vi "Sort.vi"(11 "ProgramData":T1={"Tytuły"=[], "Folder"=path "", "Data/tytul"=[], "Ostatni index"=-10, "Title"="", "Note"=""}) -> (3 "ProgramData Exit":T1={"Tytuły"=[], "Folder"=path "", "Data/tytul"=[], "Ostatni index"=-10, "Title"="", "Note"=""})   [LabVIEW 2020]
uses:
  #typeDef_ProgramData.ctl
panel:
  in  "D.Rosnąco":bool
  in  "D.Malejąco":bool
  in  "N.Rosnąco":bool
  in  "N.Malejąco":bool
  # "Sort"
  # "By name"
  # "By date"
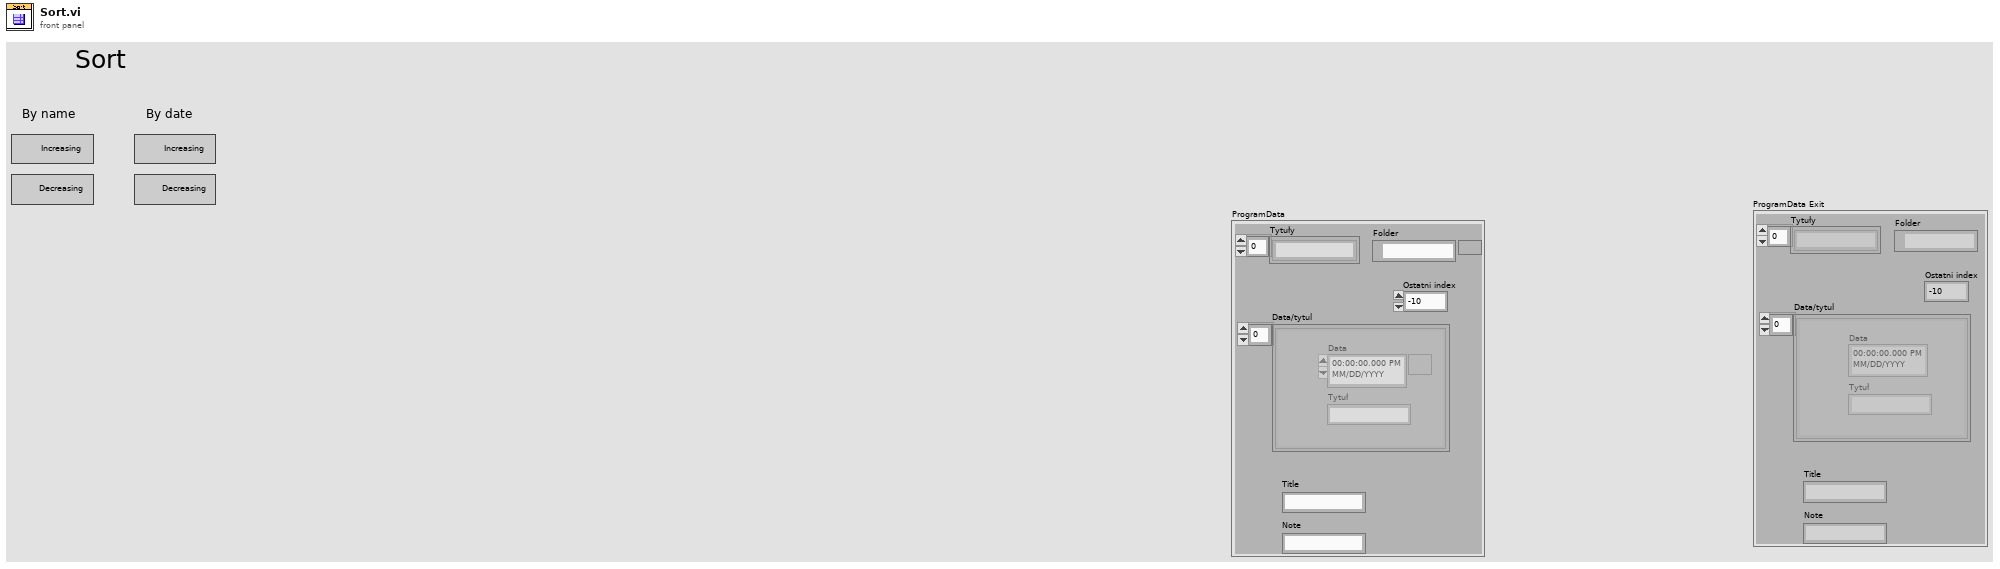
[diagram p1: front panel]
types:
  T1 = typedef "#typeDef_ProgramData.ctl" = cluster{"Tytuły":string[], "Folder":path, "Data/tytul":cluster{"Data":timestamp, "Tytuł":string}[], "Ostatni index":i32, "Title":string, "Note":string}
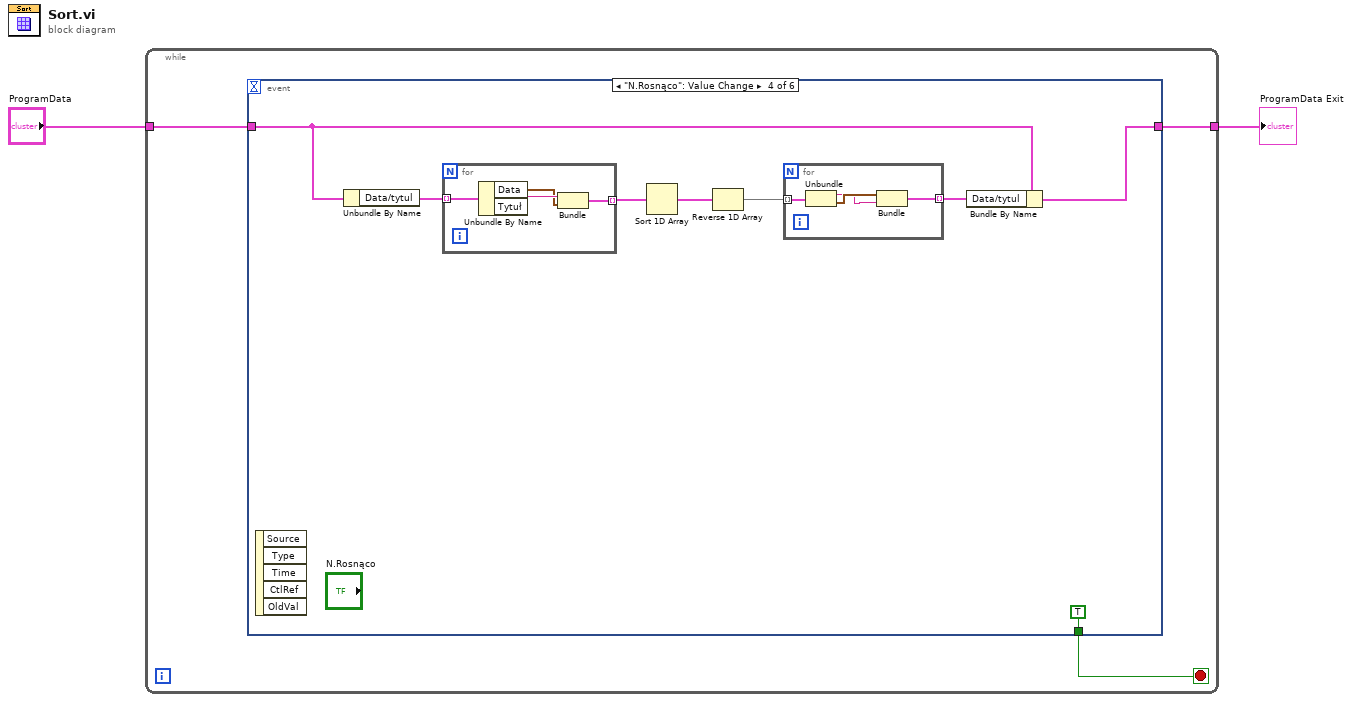
[diagram p0: block diagram]
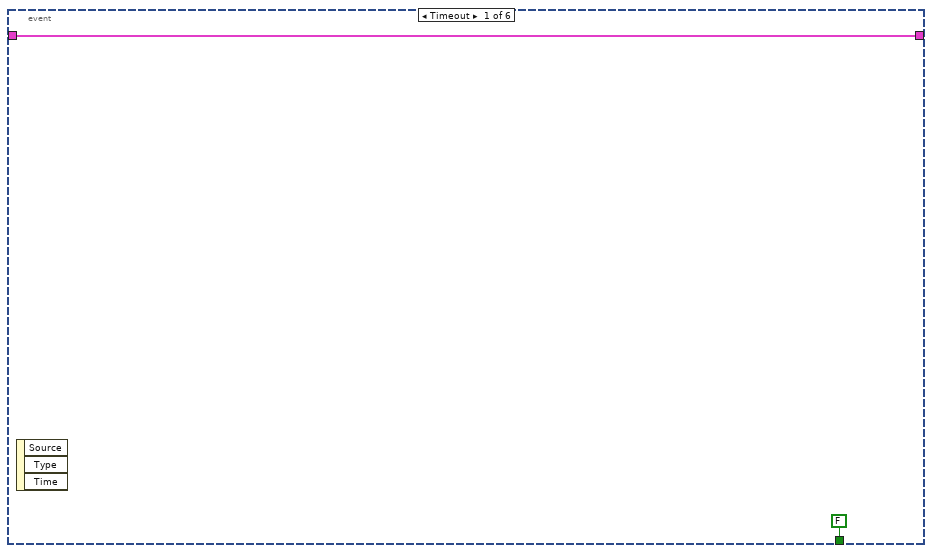
[diagram p2: hidden frame]
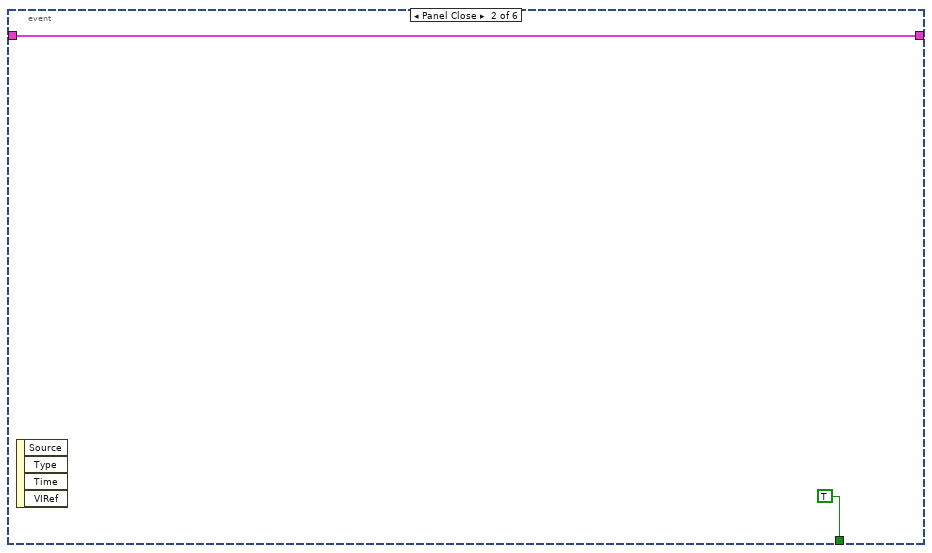
[diagram p3: hidden frame]
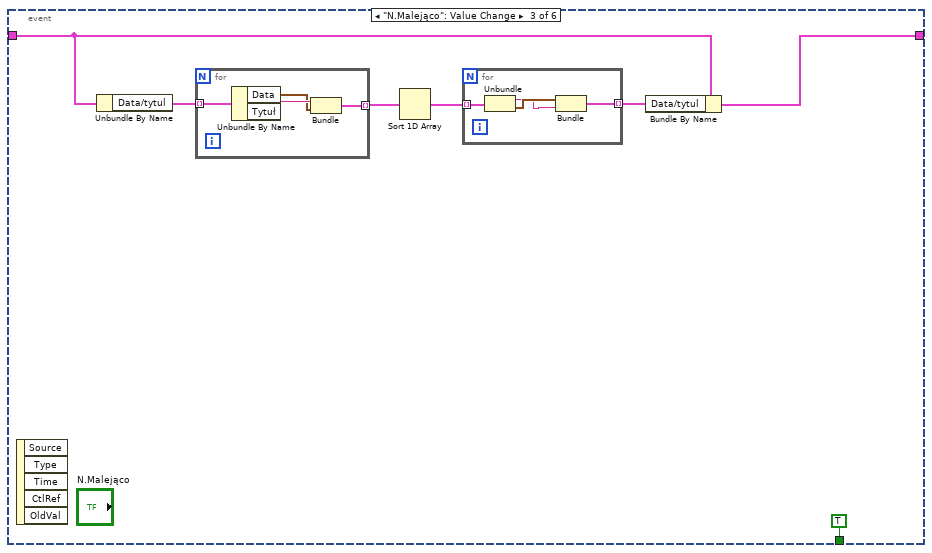
[diagram p4: hidden frame]
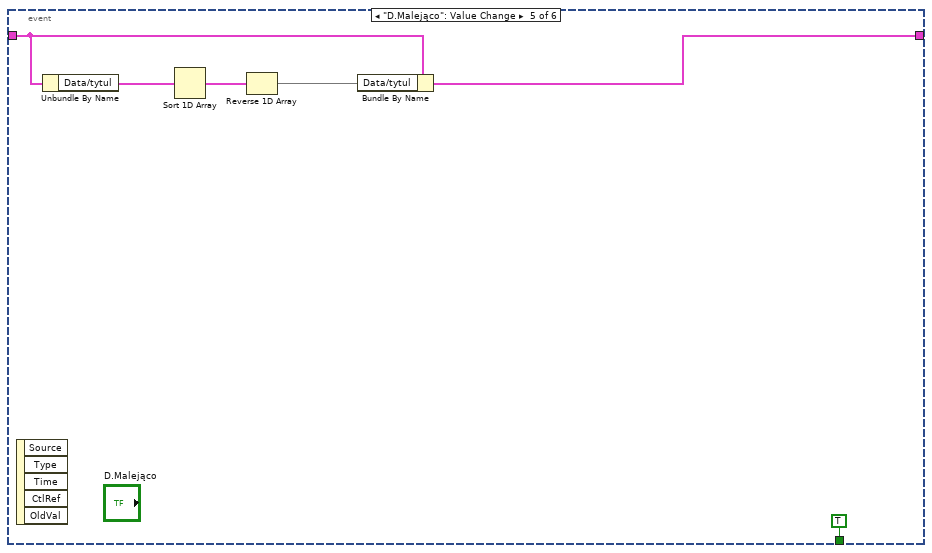
[diagram p5: hidden frame]
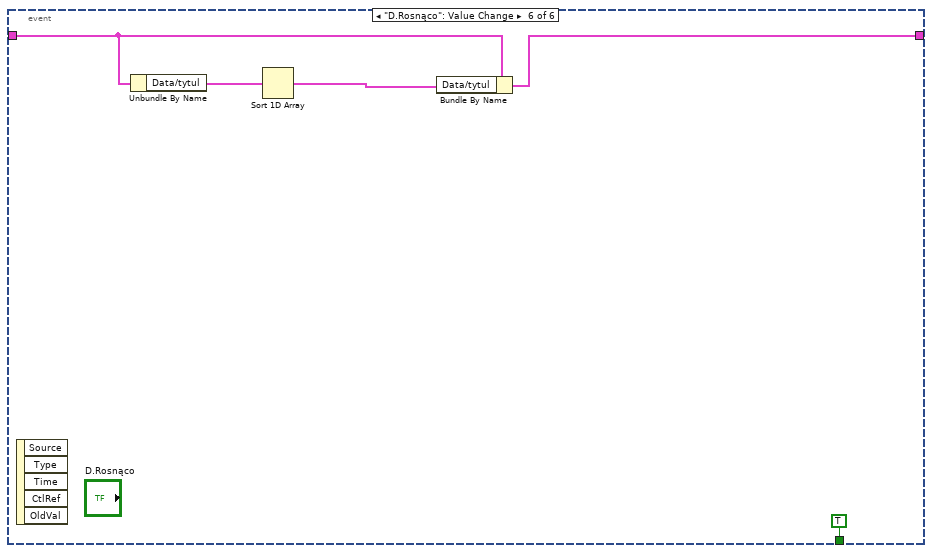
[diagram p6: hidden frame]
diagram:
  n1 = while {
    tunnel: "ProgramData" -> [w5]
    tunnel: [w4] -> w1
    stop <- w3 stop-if-true
    n2 = event shown="[3] \"N.Rosnąco\": Value Change" {
      selector: _ -> [_ _ _ _ _ _]
      dyn-events: _ -> [_ _ _ _ _ _]
      timeout: _ -> [_ _ _ _ _ _]
      tunnel: [w7 w9 w11 w26 w44 w49] -> w4
      tunnel: w5 -> [w7 w9 w14 w27 w45 w50]
      tunnel: [FALSE TRUE TRUE TRUE TRUE TRUE] -> w3
      event Timeout {
        n3 = event-data() -> ()  [unwired: 1 in, 3 out]
      }
      event Panel Close {
        n4 = event-data() -> ()  [unwired: 1 in, 4 out]
      }
      event "N.Malejąco": Value Change {
        n5 = event-data() -> ()  [unwired: 1 in, 5 out]
        n6 = Unbundle By Name(w14) -> ("Data/tytul"=w16:cluster{"Data":timestamp, "Tytuł":string}[])
        n7 = for {
          tunnel: w16 -> [w24] mode=indexing
          tunnel: [w21] -> w15 mode=indexing
          n8 = Unbundle By Name(w24) -> ("Data"=w22:timestamp, "Tytuł"=w23:string)
          n9 = Bundle("Tytuł"=w23, "Data"=w22) -> (w21:cluster{"Tytuł":string, "Data":timestamp})  [unwired: 1 in]
        }
        n10 = Sort 1D Array(array=w15) -> (sorted array=w13:cluster{"Tytuł":string, "Data":timestamp}[])
        n11 = for {
          tunnel: w13 -> [w20] mode=indexing
          tunnel: [w17] -> w12 mode=indexing
          n12 = Unbundle(w20) -> ("Tytuł"=w18:string, "Data"=w19:timestamp)
          n13 = Bundle("Data"=w19, "Tytuł"=w18) -> (w17:cluster{"Data":timestamp, "Tytuł":string})  [unwired: 1 in]
        }
        n14 = Bundle By Name(cluster=w14, "Data/tytul"=w12) -> (w11:T1)
      }
      event "N.Rosnąco": Value Change {
        n15 = event-data() -> ()  [unwired: 1 in, 5 out]
        n16 = Unbundle By Name(w27) -> ("Data/tytul"=w32:cluster{"Data":timestamp, "Tytuł":string}[])
        n17 = for {
          tunnel: w32 -> [w40] mode=indexing
          tunnel: [w37] -> w31 mode=indexing
          n18 = Unbundle By Name(w40) -> ("Data"=w38:timestamp, "Tytuł"=w39:string)
          n19 = Bundle("Tytuł"=w39, "Data"=w38) -> (w37:cluster{"Tytuł":string, "Data":timestamp})  [unwired: 1 in]
        }
        n20 = Sort 1D Array(array=w31) -> (sorted array=w30:cluster{"Tytuł":string, "Data":timestamp}[])
        n21 = Reverse 1D Array(array=w30) -> (reversed array=w28:cluster{"Tytuł":string, "Data":timestamp}[])
        n22 = for {
          tunnel: w28 -> [w36] mode=indexing
          tunnel: [w33] -> w29 mode=indexing
          n23 = Unbundle(w36) -> ("Tytuł"=w34:string, "Data"=w35:timestamp)
          n24 = Bundle("Data"=w35, "Tytuł"=w34) -> (w33:cluster{"Data":timestamp, "Tytuł":string})  [unwired: 1 in]
        }
        n25 = Bundle By Name(cluster=w27, "Data/tytul"=w29) -> (w26:T1)
      }
      event "D.Malejąco": Value Change {
        n26 = event-data() -> ()  [unwired: 1 in, 5 out]
        n27 = Unbundle By Name(w45) -> ("Data/tytul"=w46:cluster{"Data":timestamp, "Tytuł":string}[])
        n28 = Sort 1D Array(array=w46) -> (sorted array=w42:cluster{"Data":timestamp, "Tytuł":string}[])
        n29 = Reverse 1D Array(array=w42) -> (reversed array=w41:cluster{"Data":timestamp, "Tytuł":string}[])
        n30 = Bundle By Name(cluster=w45, "Data/tytul"=w41) -> (w44:T1)
      }
      event "D.Rosnąco": Value Change {
        n31 = event-data() -> ()  [unwired: 1 in, 5 out]
        n32 = Unbundle By Name(w50) -> ("Data/tytul"=w51:cluster{"Data":timestamp, "Tytuł":string}[])
        n33 = Sort 1D Array(array=w51) -> (sorted array=w47:cluster{"Data":timestamp, "Tytuł":string}[])
        n34 = Bundle By Name(cluster=w50, "Data/tytul"=w47) -> (w49:T1)
      }
    }
  }
  "ProgramData Exit" <- w1
